vi "BuildType.vi"(10 "Tag":string, 11 "Value":string) -> (3 "XML":string)   [LabVIEW 2013]
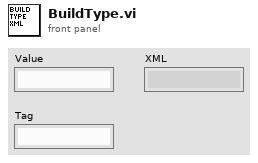
[diagram p1: front panel]
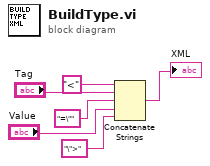
[diagram p0: block diagram]
diagram:
  n1 = Concatenate Strings("<" ("string"), "Tag", "=\"" ("string"), "Value", "\">" ("string")) -> (→"XML":string)
